vi "GetVariableField.vi"(10 "Field":refnum<k24>, 11 "error in (no error)":errorcluster) -> (2 "Field cluster":T1, 3 "error out":errorcluster)   [LabVIEW 2011, in "UnderAutomation.Fanuc.lvlib"]
uses:
  UnderAutomation.Fanuc.lvlib
  C:/Users/fg/Documents/Fanuc.vi/LabVIEW_2024/UnderAutomation.Fanuc/lib/UnderAutomation.Fanuc.dll
  LabVIEW_2024/UnderAutomation.Fanuc/lib/UnderAutomation.Fanuc.dll
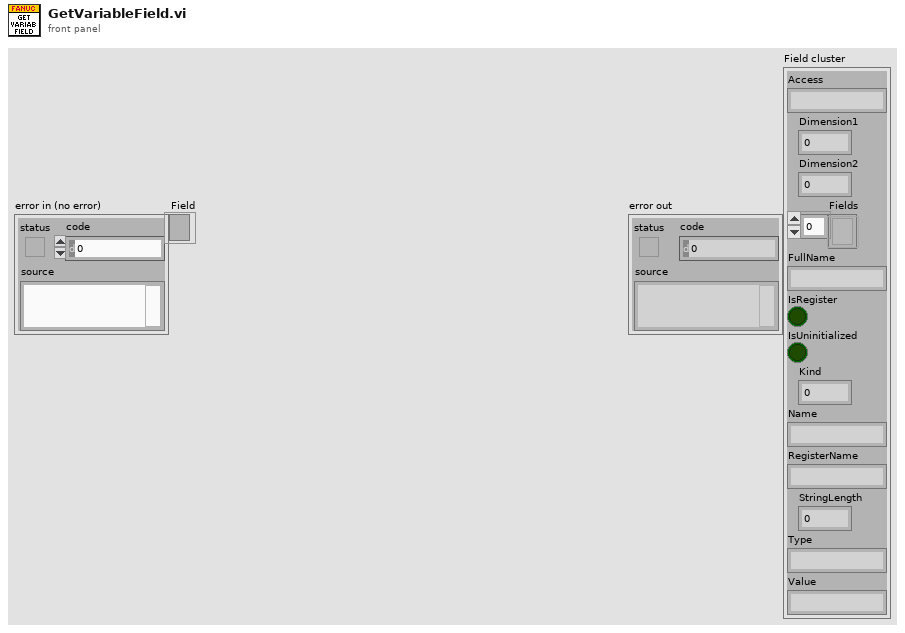
[diagram p1: front panel]
types:
  T1 = cluster{"Access":string, "Dimension1":i32, "Dimension2":i32, "Fields":refnum<k24>[], "FullName":string, "IsRegister":bool, "IsUninitialized":bool, "Kind":i32, "Name":string, "RegisterName":string, "StringLength":i32, "Type":string, "Value":string}
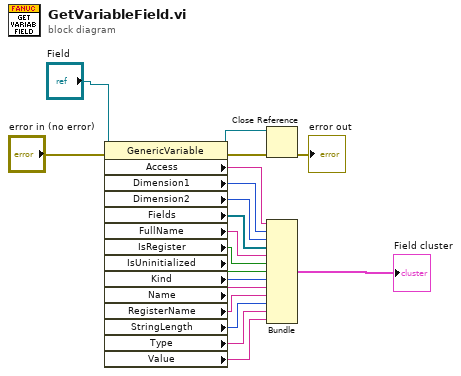
[diagram p0: block diagram]
diagram:
  n1 = property class="GenericVariable"(reference="Field", error in="error in (no error)") -> (reference out=w2:refnum<k24>, error out=w4:errorcluster, "Access"=w19:string, "Dimension1"=w18:i32, "Dimension2"=w17:i32, "Fields"=w16:refnum<k24>[], "FullName"=w15:string, "IsRegister"=w14:bool, "IsUninitialized"=w13:bool, "Kind"=w12:i32, "Name"=w11:string, "RegisterName"=w10:string, "StringLength"=w9:i32, "Type"=w8:string, "Value"=w7:string)
  n2 = Close Reference(reference=w2, error in (no error)=w4) -> (error out=→"error out":errorcluster)
  n3 = Bundle("Access"=w19, "Dimension1"=w18, "Dimension2"=w17, "Fields"=w16, "FullName"=w15, "IsRegister"=w14, "IsUninitialized"=w13, "Kind"=w12, "Name"=w11, "RegisterName"=w10, "StringLength"=w9, "Type"=w8, "Value"=w7) -> (→"Field cluster":T1)  [unwired: 1 in]
